vi "Create dbTable if not exist.vi"(4 "flatten cluster? (f)":bool, 5 "Max string size(30)":i32=30, 6 "data":variant, 7 "use file? (f)":bool, 8 "error in (no error)":errorcluster, 9 "columns":string[](array[string]), 10 "table name":string, 11 "connection reference":T1) -> (0 "error out":errorcluster, 1 "columns out":string[](array[string]), 2 "table name out":string, 3 "connection reference out":T1)   [LabVIEW 2013, in "Database Lib.lvlib"]
doc: "Creates a new table in the database identified by <B>connection reference</B> if that table does not already exist. The <B>table name</B>, <B>columns</B>, and <B>parameters</B> inputs describe the name of the table, the names of the columns (fields), and the parameter properties of each column, respectively."
uses:
  Database Lib.lvlib
  Utility/database/Connection.llb/Conn ObjectReference.ctl
  Utility/database/Auxilliary.llb/DB Tools Column Info.ctl
  Utility/database/Auxilliary.llb/DB Tools DataTypes.ctl
  Utility/database/NI_Database_API_64.lvlib
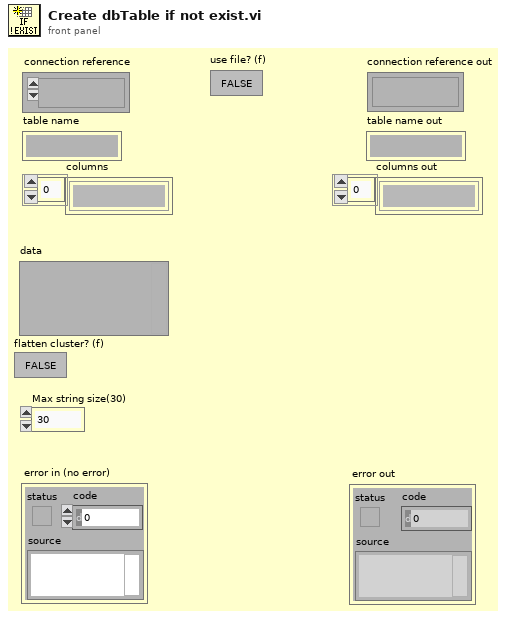
[diagram p1: front panel]
types:
  T1 = typedef "NI_Database_API_64.lvlib/Conn ObjectReference.ctl" = refnum<k1>
  T2 = typedef "NI_Database_API_64.lvlib/DB Tools Parameter Info.ctl" = cluster{"parameter name":string, "type":T3, "direction":T4, "value":variant}
  T3 = typedef "NI_Database_API_64.lvlib/DB Tools DataTypes.ctl" = enum16{"String", "Long (I32)", "Single (SGL)", "Double (DBL)", "Date/Time", "Binary"}
  T4 = typedef "NI_Database_API_64.lvlib/DB Tools Parameter Dir.ctl" = enum32{"Input", "Output", "Input/Output", "Return Value"}
  T5 = typedef "NI_Database_API_64.lvlib/DB Tools Column Info.ctl" = cluster{"column name":string, "data type":T3, "size":i32, "allow null?":bool}
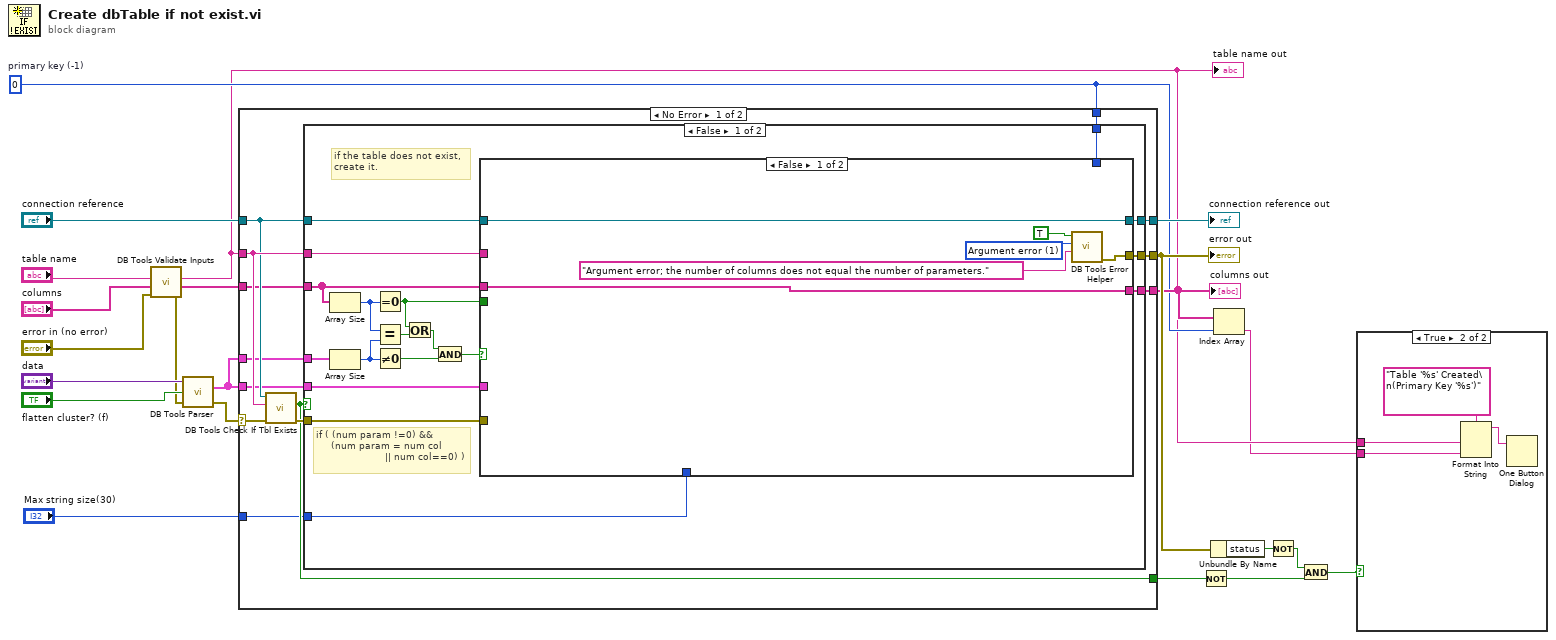
[diagram p0: block diagram]
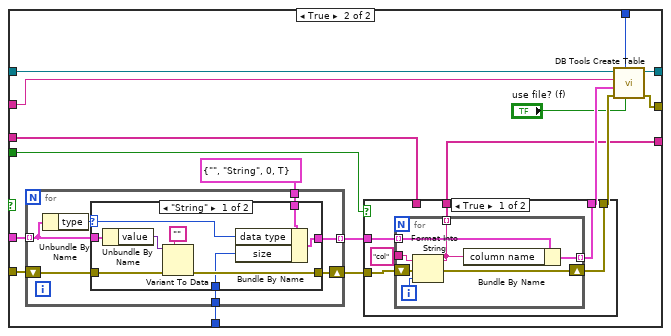
[diagram p3: hidden frame]
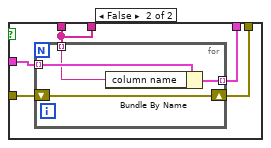
[diagram p4: hidden frame]
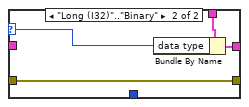
[diagram p5: hidden frame]
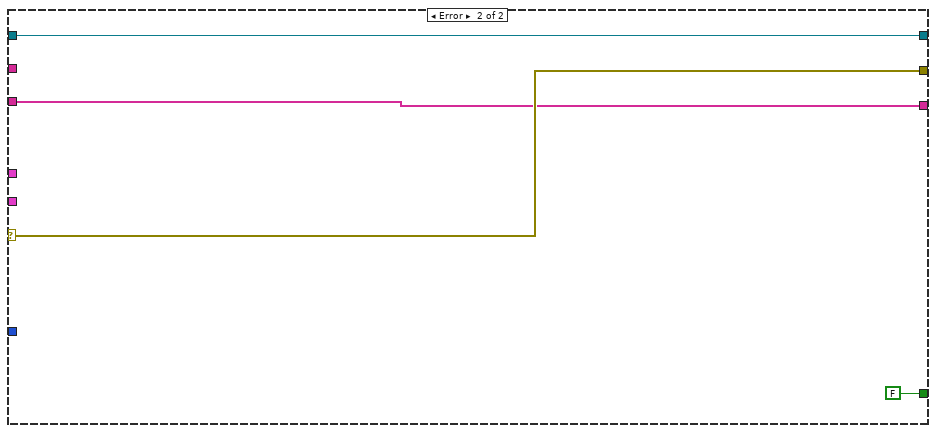
[diagram p7: hidden frame]
diagram:
  w5 = 0  # primary key (-1)
  n1 = call "DB Tools Validate Inputs.vi"("error in (no error)"="error in (no error)", "columns"="columns", "table"="table name") -> ("error out"=w18:errorcluster, "columns out"=w13:string[], "table out"=w4:string)  [unwired: 2 out]
  "table name out" <- w4
  n2 = call "DB Tools Parser.vi"("error in (no error)"=w18, "flatten cluster? (F)"="flatten cluster? (f)", "variant"="data") -> ("error out"=w15:errorcluster, "parameters"=w14:T2[])  [unwired: 1 out]
  n3 = case shown="No Error" w15 {
    selector: w15 -> [w35 w125]
    tunnel: "connection reference" -> [w30 w124]
    tunnel: w4 -> [w33 _]
    tunnel: [w32 w125] -> w9
    tunnel: [w31 w124] -> w21
    tunnel: w14 -> [w29 _]
    tunnel: w13 -> [w28 w123]
    tunnel: w14 -> [w27 _]
    tunnel: [w26 w123] -> w6
    tunnel: [w25 FALSE ("exists?")] -> w11
    tunnel: w5 -> [w24 _]
    tunnel: "Max string size(30)" -> [w23 _]
    frame No Error {
      n4 = call "DB Tools Check If Tbl Exists.vi"("error in (no error)"=w35, "table name"=w33, "connection reference"=w30) -> ("error out"=w34:errorcluster, "exists?"=w25:bool)  [unwired: 3 out]
      n5 = case shown="False" w25 {
        tunnel: w34 -> [w42 w121]
        tunnel: w33 -> [w38 _]
        tunnel: [w53 w121] -> w32
        tunnel: [w52 w120] -> w31
        tunnel: w30 -> [w51 w120]
        tunnel: w29 -> [w44 _]
        tunnel: w28 -> [w46 w119]
        tunnel: w27 -> [w43 _]
        tunnel: [w40 w119] -> w26
        tunnel: w24 -> [w37 _]
        tunnel: w23 -> [w36 _]
        frame False {
          # "if ( (num param !=0) &&\n     (num param = num col \n                       || num col==0) )"
          # "if the table does not exist, \ncreate it."
          n6 = Array Size(array=w46) -> (size(s)=w50:i32)
          n7 = Array Size(array=w44) -> (size(s)=w41:i32)
          n8 = Equal To 0?(x=w50) -> (x = 0?=w39:bool)
          n9 = Equal?(x=w50, y=w41) -> (x = y?=w49:bool)
          n10 = Not Equal To 0?(x=w41) -> (x != 0?=w47:bool)
          n11 = Or(x=w39, y=w49) -> (x .or. y?=w48:bool)
          n12 = And(x=w48, y=w47) -> (x .and. y?=w45:bool)
          n13 = case shown="False" w45 {
            tunnel: w38 -> [_ w76]
            tunnel: [w57 w75] -> w53
            tunnel: [w56 w74] -> w52
            tunnel: w51 -> [w56 w73]
            tunnel: w46 -> [w55 w64]
            tunnel: w43 -> [_ w72]
            tunnel: w42 -> [_ w71]
            tunnel: [w55 w66] -> w40
            tunnel: w39 -> [_ w65]
            tunnel: w37 -> [_ w61]
            tunnel: w36 -> [_ w60]
            frame False {
              w59 = 1 items=["No error", "Argument error", "Memory is full", "Out of zone", "End of file", "File already open", "Generic file I/O error", "File not found", "File permission error", "Disk is full", "Duplicate path", "Too many files open", "System feature not enabled", "Resource file not found", "Cannot add resource", "Resource not found", "Image not found", "Image memory error", "Pen does not exist", "Config type invalid", "Config token not found", "Config parse error", "Config memory error", "Bad external code format", "Bad external code offset", "External code not present", "Null window", "Destroy window error", "Null menu", "Print aborted", "Bad print record", "Print driver error", "Windows error during printing", "Memory error during printing", "Print dialog error", "Generic print error", "Invalid device refnum", "Device not found", "Device parameter error", "Device unit error", "Cannot open device", "Device call aborted", "Generic error", "Cancelled by user", "Object ID too low", "Object ID too high", "Object not in heap", "Unknown heap", "Unknown object (invalid DefProc)", "Unknown object (DefProc not in table)", "Message out of range", "Invalid (null) method", "Unknown message", "Manager call not supported", "Bad address", "Network operation in progress", "Network operation timed out", "Connection is busy", "Network attribute not supported", "Network error", "Address in use", "System out of memory", "Connection aborted", "Connection refused", "Not connected", "Already connected", "Connection closed", "Initialization error (interapplication manager)", "Bad occurrence", "Wait on unbound occurrence handler", "Occurrence queue overflow", "Datalog type conflict", "Unused", "Unrecognized type (interapplication manager)", "Memory corrupt", "Failed to make temporary DLL", "Old CIN version", "Drag socket not found", "Failed to load drop-object", "Failed to register OLE object", "Failed to release OLE object", "Format specifier type mismatch", "Unknown format specifier", "Too few format specifiers", "Too many format specifiers", "Scan failed", "Newer CIN version", "Error converting to variant", "Runtime menu error", "Password tampered", "Variant attribute not found", "Incompatible variant data type", "Event data is not available", "Event Store is not present", "Occurrence is not found", "Event Queue is not created", "Event info is not available", "Refnum passed is NULL", "Error retrieving Class GUID", "Error retrieving CoClass GUID", "Error retrieving TypeLib GUID.", "Bad built application magic bytes.", "Specific driver is different from the specific driver associated with the Logical Name.", "There is no session opened to the class driver.", "Max Error", "MAX - Error with config objects", "MAX - Error loading configuration", "MAX - Group not supported"]
              n14 = call "DB Tools Error Helper.vi"("source"="Argument error; the number of columns does not equal the number of parameters.", "code"=w59, "status"=TRUE) -> ("error out"=w57:errorcluster)  [unwired: 8 in]
            }
            frame True {
              n15 = for {
                tunnel: w72 -> [w102] mode=indexing
                shift-right: [w103] -> w63
                shift-left: w71 -> [w104]
                tunnel: T5 {"column name"="", "data type"=enum."String", "size"=0, "allow null?"=TRUE} ("column information") -> [w105]
                tunnel: [w101] -> w69 mode=indexing
                tunnel: w60 -> [w99]
                n16 = Unbundle By Name(w102) -> ("type"=w100:T3)
                n17 = case shown="\"String\"" w100 {
                  selector: w100 -> [w107 w115]
                  tunnel: [w112 w117] -> w101
                  tunnel: w102 -> [w111 _]
                  tunnel: w105 -> [w108 w116]
                  tunnel: w104 -> [w110 w118]
                  tunnel: [w109 w118] -> w103
                  tunnel: w99 -> [w106 _]
                  frame "String" {
                    n18 = Unbundle By Name(w111) -> ("value"=w114:variant)
                    n19 = Variant To Data(error in=w110, type="", Variant=w114) -> (error out=w109:errorcluster)  [unwired: 1 out]
                    n20 = Bundle By Name(cluster=w108, "data type"=w107, "size"=w106) -> (w112:T5)
                  }
                  frame "Long (I32)".."Binary" {
                    n21 = Bundle By Name(cluster=w116, "data type"=w115) -> (w117:T5)
                  }
                }
              }
              n22 = case shown="True" w65 {
                tunnel: w69 -> [w81 w94]
                tunnel: [w80 w93] -> w68
                tunnel: [w79 w92] -> w67
                tunnel: [w78 w90] -> w66
                tunnel: w64 -> [_ w90]
                tunnel: w63 -> [w77 w91]
                frame True {
                  n23 = for {
                    tunnel: "col" -> [w88]
                    shift-right: [w86] -> w79
                    shift-left: w77 -> [w87]
                    tunnel: [w85] -> w80 mode=indexing
                    tunnel: w81 -> [w84] mode=indexing
                    tunnel: [w83] -> w78 mode=indexing
                    i -> [w89]
                    n24 = Format Into String(initial string=w88, error in=w87, w89) -> (resulting string=w83:string, error out=w86:errorcluster)  [unwired: 1 in]
                    n25 = Bundle By Name(cluster=w84, "column name"=w83) -> (w85:T5)
                  }
                }
                frame False {
                  n26 = for {
                    shift-right: [w95] -> w92
                    shift-left: w91 -> [w95]
                    tunnel: [w98] -> w93 mode=indexing
                    tunnel: w94 -> [w97] mode=indexing
                    tunnel: w90 -> [w96] mode=indexing
                    n27 = Bundle By Name(cluster=w97, "column name"=w96) -> (w98:T5)
                  }
                }
              }
              n28 = call "DB Tools Create Table.vi"("use file? (F)"="use file? (f)", "primary key (-1)"=w61, "error in (no error)"=w67, "column information"=w68, "table"=w76, "connection reference"=w73) -> ("error out"=w75:errorcluster, "connection reference out"=w74:T1)  [unwired: 2 out]
            }
          }
        }
        frame True {
          # "if the table exists, the do not create it"
        }
      }
    }
    frame Error {
    }
  }
  "error out" <- w9
  "connection reference out" <- w21
  "columns out" <- w6
  n29 = Not(x=w11) -> (.not. x?=w10:bool)
  n30 = Unbundle By Name(w9) -> ("status"=w7:bool)
  n31 = Index Array(array=w6, index=w5) -> (element=w3:string)
  n32 = Not(x=w7) -> (.not. x?=w8:bool)
  n33 = And(x=w8, y=w10) -> (x .and. y?=w2:bool)
  n34 = case shown="True" w2 {
    tunnel: w4 -> [_ w128]
    tunnel: w3 -> [_ w127]
    frame False {
    }
    frame True {
      n35 = Format Into String(format string="Table '%s' Created\n(Primary Key '%s')", w128, w127) -> (resulting string=w126:string)  [unwired: 2 in, 1 out]
      n36 = One Button Dialog(message=w126) -> ()  [unwired: 2 out]
    }
  }
